vi "Configure.vi"(8 "error in (no error)":errorcluster, 10 "Network Stream Writer IP":string, 11 "DataReceiver in":refnum<class "DataReceiver.lvclass">) -> (0 "error out":errorcluster, 3 "DataReceiver out":refnum<class "DataReceiver.lvclass">)   [LabVIEW 2010, in "DataReceiver.lvclass"]
uses:
  DataReceiver.lvclass
  DataReceiver.lvclass/DataReceiver.ctl
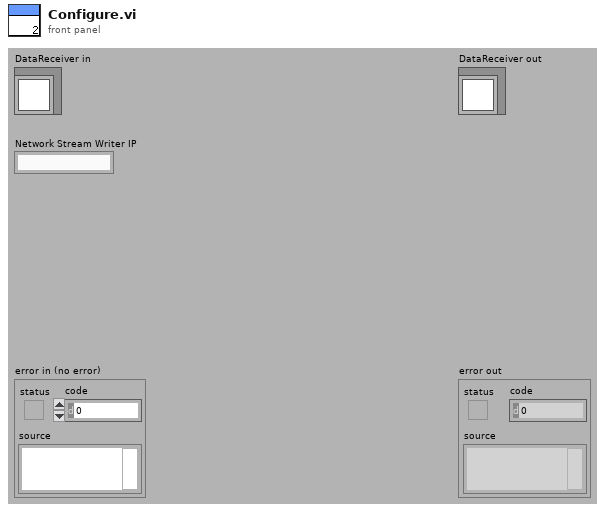
[diagram p1: front panel]
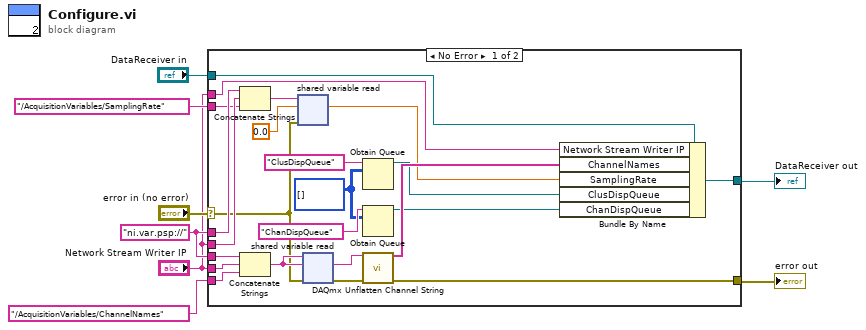
[diagram p0: block diagram]
diagram:
  w3 = "ni.var.psp://" ("string")
  n1 = case shown="No Error" "error in (no error)" {
    selector: "error in (no error)" -> [w22 w33]
    tunnel: [w10 w33] -> w7
    tunnel: [w11 w32] -> w5
    tunnel: "DataReceiver in" -> [w21 w32]
    tunnel: "Network Stream Writer IP" -> [w31 _]
    tunnel: w3 -> [w28 _]
    tunnel: "/AcquisitionVariables/ChannelNames" ("string") -> [w27 _]
    tunnel: "Network Stream Writer IP" -> [w26 _]
    tunnel: w3 -> [w25 _]
    tunnel: "/AcquisitionVariables/SamplingRate" ("string") -> [w24 _]
    tunnel: "Network Stream Writer IP" -> [w9 _]
    frame No Error {
      w14 = i32[][] []
      n2 = Concatenate Strings(w25, w26, w24) -> (w29:string)
      n3 = Concatenate Strings(w28, w31, w27) -> (w30:string)
      n4 = shared-variable-read(w29, w22, 0.0) -> (w17:dbl)  [unwired: 3 out]
      n5 = shared-variable-read(w30, w22, w30) -> (w19:errorcluster, w20:string)  [unwired: 2 out]
      n6 = Obtain Queue(name (unnamed)="ClusDispQueue", element data type=w14) -> (queue out=w13:refnum<queue>)  [unwired: 3 in, 2 out]
      n7 = Obtain Queue(name (unnamed)="ChanDispQueue", element data type=w14) -> (queue out=w12:refnum<queue>)  [unwired: 3 in, 2 out]
      n8 = call <vilib>:"DAQmx Unflatten Channel String.vi"("names in"=w20, "error in"=w19) -> ("names out"=w18:string[], "error out"=w10:errorcluster)  [unwired: 12 in]
      n9 = Bundle By Name(cluster=w21, "Network Stream Writer IP"=w9, "ChannelNames"=w18, "SamplingRate"=w17, "ClusDispQueue"=w13, "ChanDispQueue"=w12) -> (w11:refnum<class "DataReceiver.lvclass">)
    }
    frame Error {
    }
  }
  "error out" <- w7
  "DataReceiver out" <- w5
